vi "X509_get_issuer_name.vi"(8 "error in (no error)":errorcluster, 11 "X509-Cert in":refnum<class "X509-Cert.lvclass">) -> (0 "error out":errorcluster, 2 "issuer name":string, 3 "X509-Cert out":refnum<class "X509-Cert.lvclass">)   [LabVIEW 2013, in "SSL_Lib.lvlib" / "X509-Cert.lvclass"]
uses:
  X509-Cert.lvclass
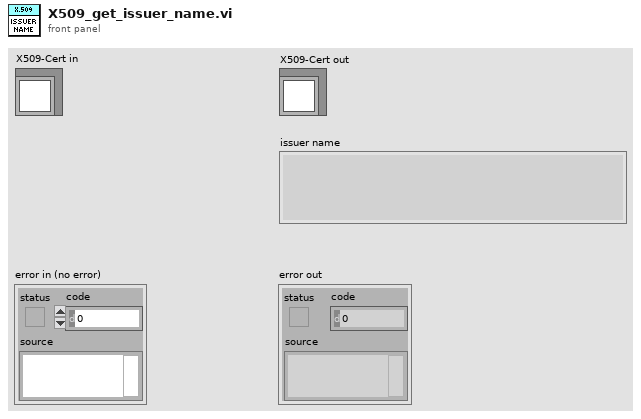
[diagram p1: front panel]
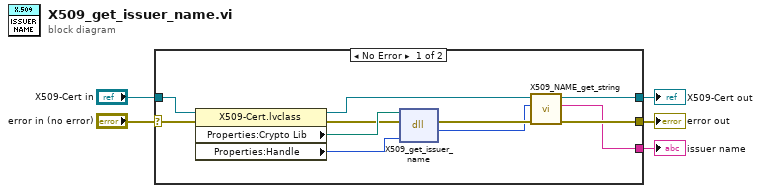
[diagram p0: block diagram]
diagram:
  n1 = case shown="No Error" "error in (no error)" {
    selector: "error in (no error)" -> [w14 w17]
    tunnel: [w10 w17] -> w4
    tunnel: "X509-Cert in" -> [w15 w16]
    tunnel: [w9 _] -> w2
    tunnel: [w6 w16] -> w1
    frame No Error {
      n2 = property class="X509-Cert.lvclass"(reference=w15, error in=w14) -> (reference out=w7:refnum<class "X509-Cert.lvclass">, error out=w11:errorcluster, "Properties:Crypto Lib"=w12:path, "Properties:Handle"=w13:u64)
      n3 = dll-call lib="C:/Program Files (x86)/National Instruments/Shared/nissl/NIlibeay32.dll" fn="X509_get_issuer_name"(path in=w12, error in=w11, "X509"=w13) -> ("return type"=w8:u64)  [unwired: 2 in, 2 out]
      n4 = call "X509_NAME_get_string.vi"("error in (no error)"=w11, "X509_Name"=w8, "X509-Cert in"=w7) -> ("error out"=w10:errorcluster, "X509 Name String"=w9:string, "X509-Cert out"=w6:refnum<class "X509-Cert.lvclass">)  [unwired: 6 in]
    }
    frame Error {
    }
  }
  "error out" <- w4
  "issuer name" <- w2
  "X509-Cert out" <- w1
